vi "Write Parent.vi"(8 "Error In":errorcluster, 10 "Parent":refnum<class "Abstract.lvclass">, 11 "Node In":refnum<class "Abstract.lvclass">) -> (0 "Error Out":errorcluster, 3 "Node Out":refnum<class "Abstract.lvclass">)   [LabVIEW 2018, in "Toolkit.lvlib" / "Nodes.lvlib" / "Abstract.lvclass"]
uses:
  Abstract.lvclass
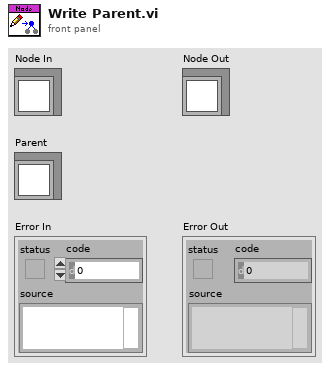
[diagram p1: front panel]
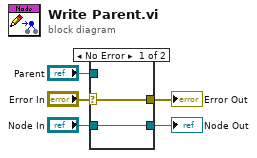
[diagram p0: block diagram]
diagram:
  n1 = case shown="No Error" "Error In" {
    selector: "Error In" -> [w7 w9]
    tunnel: [w7 w9] -> w4
    tunnel: [w6 w8] -> w1
    tunnel: "Node In" -> [w6 w8]
    tunnel: "Parent" -> [_ _]
    frame No Error {
    }
    frame Error {
    }
  }
  "Error Out" <- w4
  "Node Out" <- w1
